vi "fmt_trimFormatBuffer.vi"(8 "error in (no error)":errorcluster, 11 "format buffers in":T1) -> (0 "error out":errorcluster, 1 "max row":i32, 2 "xml":string, 3 "format buffers out":T1)   [LabVIEW 2020, in "NI_ExcelFile.lvlib"]
uses:
  <vilib>/express/express shared/NI_ExcelFile/NI_ExcelFile.lvlib
  <vilib>/express/express shared/NI_ExcelFile/Ctrls/fmt_formatBuffer.ctl
  <vilib>/express/express shared/NI_ExcelFile/Ctrls/TimeColumnMode.ctl
  <vilib>/express/express shared/NI_ExcelFile/Ctrls/Columns.ctl
  <vilib>/express/express shared/NI_ExcelFile/Ctrls/ColumnInfo.ctl
  <vilib>/express/express shared/NI_ExcelFile/Ctrls/DataType.ctl
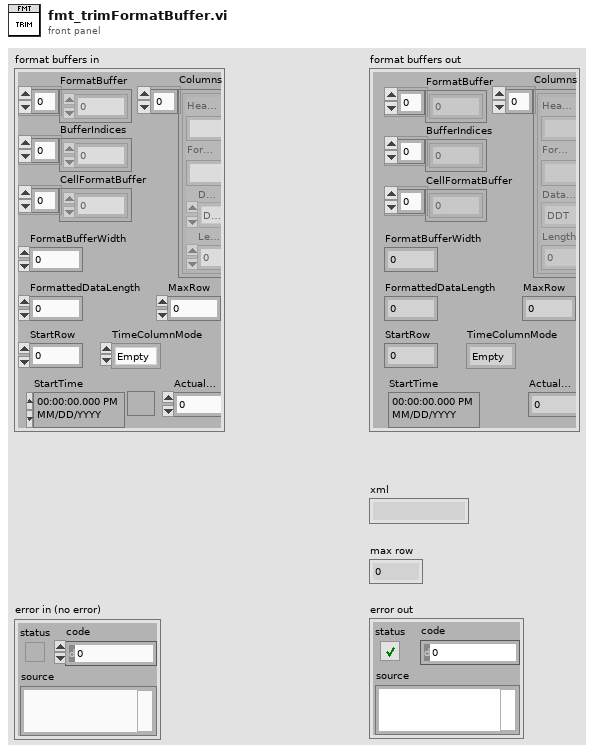
[diagram p1: front panel]
types:
  T1 = typedef "NI_ExcelFile.lvlib/fmt_formatBuffer.ctl" = cluster{"FormatBuffer":u8[], "BufferIndices":i32[], "CellFormatBuffer":u8[], "FormatBufferWidth":i32, "FormattedDataLength":i32, "MaxRow":i32, "StartRow":i32, "TimeColumnMode":T2, "StartTime":timestamp, "Columns":T3, "ActualLength":i32}
  T2 = typedef "NI_ExcelFile.lvlib/TimeColumnMode.ctl" = enum16{"Empty", "OnePerCh", "One"}
  T3 = typedef "NI_ExcelFile.lvlib/Columns.ctl" = T4[]
  T4 = typedef "NI_ExcelFile.lvlib/ColumnInfo.ctl" = cluster{"Header":string, "Format":string, "DataType":T5, "Length":u64}
  T5 = typedef "NI_ExcelFile.lvlib/DataType.ctl" = enum16{"DDT", "WFM", "Array of STR", "Array of DBL", "Array of I8", "Array of I16", "Array of I32", "Array of I64", "Array of SGL", "Array of U8", "Array of U16", "Array of U32", "Array of U64", "Array of Time"}
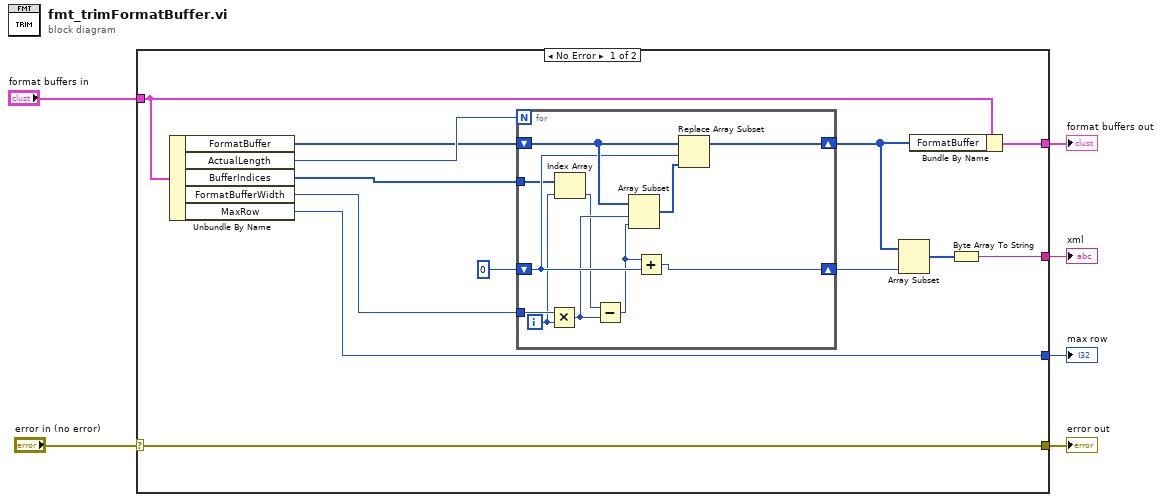
[diagram p0: block diagram]
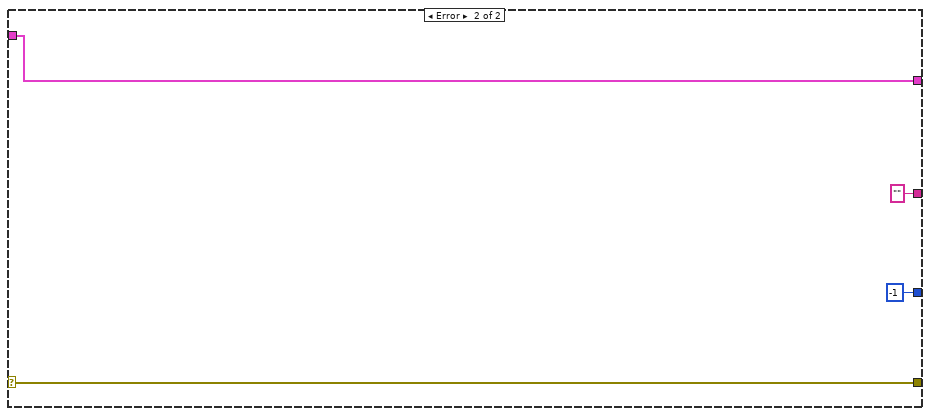
[diagram p2: hidden frame]
diagram:
  n1 = case shown="No Error" "error in (no error)" {
    selector: "error in (no error)" -> [w10 w31]
    tunnel: "format buffers in" -> [w19 w34]
    tunnel: [w18 w34] -> w5
    tunnel: [w13 "" ("string")] -> w4
    tunnel: [w11 -1 ("Max rows")] -> w3
    tunnel: [w10 w31] -> w1
    frame No Error {
      n2 = Unbundle By Name(w19) -> ("FormatBuffer"=w7:u8[], "ActualLength"=w8:i32, "BufferIndices"=w9:i32[], "FormatBufferWidth"=w16:i32, "MaxRow"=w11:i32)
      n3 = for {
        N: w8 -> [_]
        shift-right: [w30] -> w12
        shift-left: w7 -> [w29]
        shift-right: [w26] -> w15
        shift-left: 0 -> [w27]
        tunnel: w16 -> [w25]
        tunnel: w9 -> [w22]
        i -> [w21]
        n4 = Multiply(x=w25, y=w21) -> (x*y=w24:i32)
        n5 = Index Array(array=w22, index=w21) -> (element=w20:i32)
        n6 = Subtract(x=w20, y=w24) -> (x-y=w23:i32)
        n7 = Array Subset(array=w29, index=w24, length=w23) -> (w28:u8[])
        n8 = Add(x=w23, y=w27) -> (x+y=w26:i32)
        n9 = Replace Array Subset(array=w29, new element=w28, index=w27) -> (w30:u8[])
      }
      n10 = Array Subset(array=w12, length=w15) -> (w14:u8[])  [unwired: 1 in]
      n11 = Bundle By Name(cluster=w19, "FormatBuffer"=w12) -> (w18:T1)
      n12 = Byte Array To String(unsigned byte array=w14) -> (string=w13:string)
    }
    frame Error {
    }
  }
  "format buffers out" <- w5
  "xml" <- w4
  "max row" <- w3
  "error out" <- w1
